vi "Calculate Temperature Measurement Frequency.vi"(8 "error in":errorcluster, 11 "Signal In":waveform(dbl)) -> (0 "error out":errorcluster, 1 "Temperature Measurement Frequency (Seconds)":dbl, 2 "Peak Times":dbl[](array[numeric]), 3 "Peak Locations":dbl[](array[numeric]) format="%.2p")   [LabVIEW 2010]
uses:
  <vilib>/measure/mamon.llb/Waveform Peak Detection for 1 Chan.vi
  <vilib>/measure/NI_MAPro.lvlib
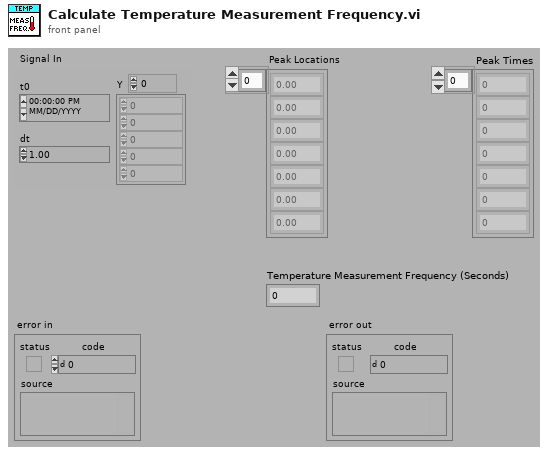
[diagram p1: front panel]
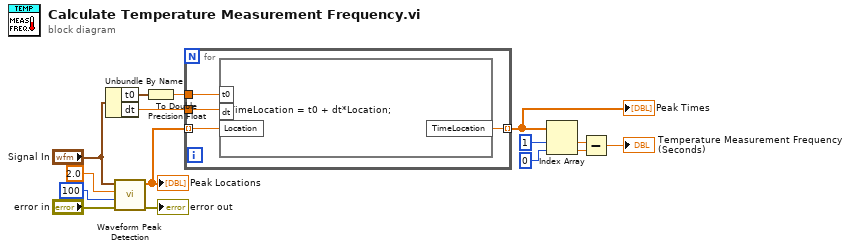
[diagram p0: block diagram]
diagram:
  n1 = Unbundle By Name("Signal In") -> ("t0"=w11:timestamp, "dt"=w9:dbl)
  n2 = call-poly <vilib>:"Waveform Peak Detection.vi"("error in"="error in", "width"=100, "threshold"=2.0, "Signal In"="Signal In") -> ("error out"=→"error out":errorcluster, "Locations"=w13:dbl[])  [unwired: 3 in, 3 out]
  "Peak Locations" <- w13
  n3 = To Double Precision Float(number=w11) -> (double precision float=w10:dbl)
  n4 = for {
    tunnel: w13 -> [w19] mode=indexing
    tunnel: w10 -> [w18]
    tunnel: w9 -> [w17]
    tunnel: [w16] -> w8 mode=indexing
    n5 = formula code="TimeLocation = t0 + dt*Location;"("Location"=w19, "t0"=w18, "dt"=w17) -> ("TimeLocation"=w16:dbl)
  }
  "Peak Times" <- w8
  n6 = Index Array(array=w8, index #1=1 ("index"), index #2=0 ("index")) -> (element #1=w4:dbl, element #2=w5:dbl)
  n7 = Subtract(x=w4, y=w5) -> (x-y=→"Temperature Measurement Frequency (Seconds)":dbl)
